vi "Remove Line.vi"(8 "error in (no error)":errorcluster, 10 "Lines to Delete":i32[](array[numeric]), 11 "Game Engine in":refnum<class "Game Engine.lvclass">) -> (0 "error out":errorcluster, 3 "Game Engine out":refnum<class "Game Engine.lvclass">)   [LabVIEW 2017, in "Game Engine.lvlib" / "Game Engine.lvclass"]
uses:
  Game Engine.lvclass
  Game Engine.lvclass/Game Engine.ctl
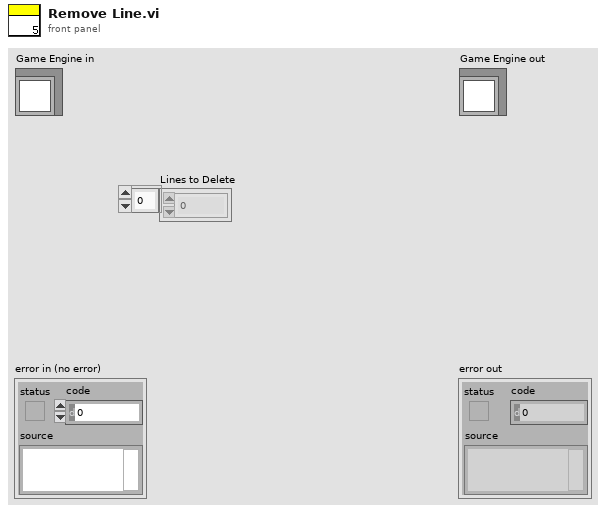
[diagram p1: front panel]
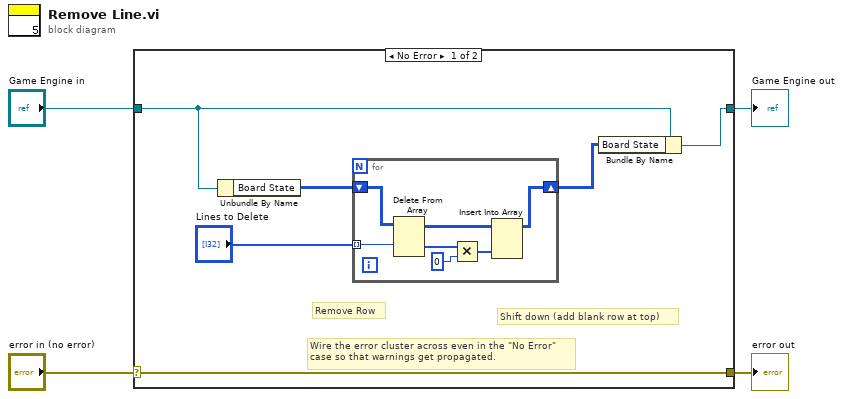
[diagram p0: block diagram]
diagram:
  n1 = case shown="No Error" "error in (no error)" {
    selector: "error in (no error)" -> [w10 w19]
    tunnel: [w10 w19] -> w3
    tunnel: [w5 w18] -> w1
    tunnel: "Game Engine in" -> [w7 w18]
    frame No Error {
      # "Shift down (add blank row at top)"
      # "Remove Row"
      # "Wire the error cluster across even in the \"No Error\"\ncase so that warnings get propagated."
      n2 = Unbundle By Name(w7) -> ("Board State"=w8:u32[][])
      n3 = for {
        tunnel: "Lines to Delete" -> [w17] mode=indexing
        shift-right: [w11] -> w6
        shift-left: w8 -> [w16]
        n4 = Delete From Array(array=w16, index (row)=w17) -> (deleted portion=w14:u32[], array with subset deleted=w15:u32[][])  [unwired: 2 in]
        n5 = Multiply(x=w14, y=0) -> (x*y=w12:u32[])
        n6 = Insert Into Array(array=w15, new element=w12) -> (w11:u32[][])  [unwired: 2 in]
      }
      n7 = Bundle By Name(cluster=w7, "Board State"=w6) -> (w5:refnum<class "Game Engine.lvclass">)
    }
    frame Error {
    }
  }
  "error out" <- w3
  "Game Engine out" <- w1
